vi "Unpack for gRPC.vi"(8 "error in":errorcluster, 9 "configuration / results":enum16{"Configuration", "Results"}(ring), 10 "any":T1, 11 "measurement plugin in":refnum<class "FPT Pulse Measurement.lvclass">) -> (0 "error out":errorcluster, 2 "data value":variant, 3 "measurement plugin out":refnum<class "FPT Pulse Measurement.lvclass">)   [LabVIEW 2023, in "FPT Pulse Measurement.lvclass"]
uses:
  FPT Pulse Measurement.lvclass
  <vilib>/gRPC/LabVIEW gRPC Library/Shared/Any.ctl
  Measurement Configuration.ctl
  Measurement Results.ctl
  a521b266-ce99-437c-923d-067dcf1e07fd.vi
  3ecd018e-d556-4cbc-bc60-c4ba57204520.vi
  <vilib>/gRPC/LabVIEW gRPC Library/Server API/Translate Protobuf Error.vi
  <vilib>/AdvancedString/1D String Array to Delimited String.vi
  <vilib>/gRPC/LabVIEW gRPC Library/Server API/Server/Get Server DLL Path.vi
  FPT Pulse Measurement.lvclass/FPT Pulse Measurement.ctl
  <vilib>/Plug-In SDKs/Measurements/Measurement Plugin Service/Measurement Plugin Service.lvclass
  <vilib>/gRPC/LabVIEW gRPC Library/grpc-lvsupport-release.lvlib
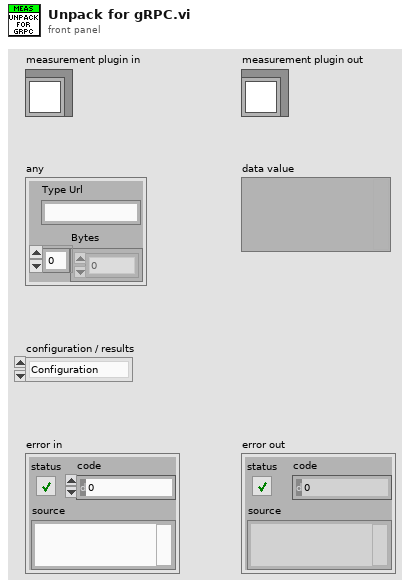
[diagram p1: front panel]
types:
  T1 = typedef "grpc-lvsupport-release.lvlib/Any.ctl" = cluster{"Type Url":string, "Bytes":u8[]}
  T2 = typedef "grpc-lvsupport-release.lvlib/grpcId.ctl" = u64
  T3 = typedef "FPT Pulse Measurement.lvclass/Measurement Configuration.ctl" = cluster{"Automation Test":bool, "Power sequencing file path":string, "RFSG name":string, "RFSG port":string, "RFSG attenuation mode":enum32{"<None>", "Constant Attenuation", "s2p File"}, "RFSG external attenuation (dB)":dbl, "RFSG s-parameters orientation":enum32{"Port1 Towards DUT", "Port2 Towards DUT"}, "RFSG s2p file path":string, "RFmx name":string, "RFmx port":string, "RFmx attenuation mode":enum32{"<None>", "Constant Attenuation", "s2p File"}, "RFmx external attenuation (dB)":dbl, "RFmx s-parameters orientation":enum32{"Port1 Towards DUT", "Port2 Towards DUT"}, "RFmx s2p file path":string, "RFmx Center Frequency (Hz)":dbl, "RFmx Measurement Bandwidth (Hz)":dbl, "RFmx Reference Level (dBm)":dbl, "RFSG Generation IQ Rate (S/s)":dbl, "Pulse Acquisition Length (s)":dbl, "Pulse Power Level (dBm)":dbl, "Pulse Repetition Interval [PRI] (s)":dbl, "Pulse Width (s)":dbl, "Number of Pulses per Burst":u32, "Measurement Offset":i32, "Window Start (%)":dbl, "Window Stop (%)":dbl, "Window Step Size (%)":dbl, "High Reference Level (%)":dbl, "Width Reference Level (%)":dbl, "Low Reference Level (%)":dbl, "Selected Pulse Trace":i32, "Power sequencing file validity check":bool}
  T4 = typedef "FPT Pulse Measurement.lvclass/Measurement Results.ctl" = cluster{"Status":string, "TS Intrapulse Stability":dbl[][], "TS P2P Stability":dbl[][], "TS Acquired Amplitude":dbl[][], "Per Pulse Result":dbl[][], "Per Pulse Result (Name)":string[], "Duty Cycle (%)":dbl, "Rising Time (us)":dbl, "Fall Time (us)":dbl, "Droop (%)":dbl, "Ripple (%)":dbl, "Overshoot (%)":dbl, "Amplitude Stability (dB)":dbl, "Phase Stability (dB)":dbl}
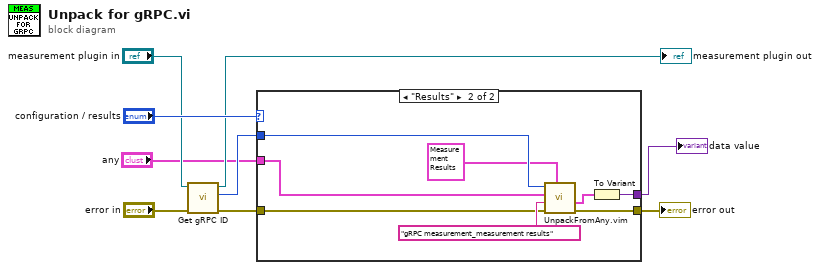
[diagram p0: block diagram]
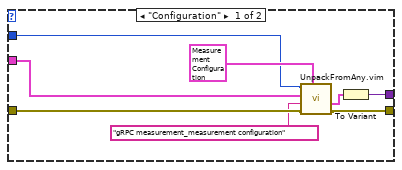
[diagram p2: hidden frame]
diagram:
  n1 = call <vilib>:"Get gRPC ID.vi"("error in"="error in", "measurement plugin service in"="measurement plugin in") -> ("error out"=w6:errorcluster, "gRPC ID"=w3:T2, "measurement plugin service out"=→"measurement plugin out":refnum<class "FPT Pulse Measurement.lvclass">)  [unwired: 7 in]
  n2 = case shown="\"Results\"" "configuration / results" {
    tunnel: w6 -> [w15 w19]
    tunnel: "any" -> [w10 w18]
    tunnel: w3 -> [w12 w22]
    tunnel: [w16 w23] -> w9
    tunnel: [w17 w25] -> w1
    frame "Configuration" {
      n3 = call "UnpackFromAny.vim"("Data Type"=T3 {"Automation Test"=FALSE, "Power sequencing file path"="Lorem ipsum dolor sit", "RFSG name"="5842_0", "RFSG port"="", "RFSG attenuation mode"=enum."s2p File", "RFSG external attenuation (dB)"=-32.0, "RFSG s-parameters orientation"=enum."Port1 Towards DUT", "RFSG s2p file path"="", "RFmx name"="5842_0", "RFmx port"="", "RFmx attenuation mode"=enum."Constant Attenuation", "RFmx external attenuation (dB)"=1.0, "RFmx s-parameters orientation"=enum."Port1 Towards DUT", "RFmx s2p file path"="", "RFmx Center Frequency (Hz)"=10000000000.0, "RFmx Measurement Bandwidth (Hz)"=80000000.0, "RFmx Reference Level (dBm)"=10.0, "RFSG Generation IQ Rate (S/s)"=1250000000.0, "Pulse Acquisition Length (s)"=0.001, "Pulse Power Level (dBm)"=-20.0, "Pulse Repetition Interval [PRI] (s)"=0.0001, "Pulse Width (s)"=2e-05, "Number of Pulses per Burst"=20, "Measurement Offset"=0, "Window Start (%)"=10.0, "Window Stop (%)"=90.0, "Window Step Size (%)"=10.0, "High Reference Level (%)"=90.0, "Width Reference Level (%)"=50.0, "Low Reference Level (%)"=10.0, "Selected Pulse Trace"=0, "Power sequencing file validity check"=FALSE} ("Measurement Configuration"), "error in"=w15, "Message Type"="gRPC measurement_measurement configuration", "Any"=w10, "gRPCid in"=w12) -> ("error out"=w16:errorcluster, "Unpacked Value"=w14:T3)  [unwired: 4 in, 1 out]
      n4 = To Variant(anything=w14) -> (Variant=w17:variant)
    }
    frame "Results" {
      n5 = call "UnpackFromAny.vim"("Data Type"=T4 {"Status"="Empty", "TS Intrapulse Stability"=[], "TS P2P Stability"=[], "TS Acquired Amplitude"=[], "Per Pulse Result"=[], "Per Pulse Result (Name)"=[], "Duty Cycle (%)"=0.0, "Rising Time (us)"=0.0, "Fall Time (us)"=0.0, "Droop (%)"=0.0, "Ripple (%)"=0.0, "Overshoot (%)"=0.0, "Amplitude Stability (dB)"=0.0, "Phase Stability (dB)"=0.0} ("Measurement Results"), "error in"=w19, "Message Type"="gRPC measurement_measurement results", "Any"=w18, "gRPCid in"=w22) -> ("error out"=w23:errorcluster, "Unpacked Value"=w24:T4)  [unwired: 4 in, 1 out]
      n6 = To Variant(anything=w24) -> (Variant=w25:variant)
    }
  }
  "error out" <- w9
  "data value" <- w1
